vi "WSP2_InsertProcessDataWithFails.vi"(4 "Employee":string, 5 "FailString":string, 6 "EndTime":string, 7 "EntryTime":string, 8 "PassFail":i32, 9 "ProcessName":string, 10 "StationName":string, 11 "SerialNumber":string) -> (0 "error out":errorcluster, 3 "ReplyTrace":string)   [LabVIEW 2023]
uses:
  C:/Elatch-Bench-Test/VIs 64 bits/Elatch-Bench-Test/DLL/WSConnector.dll
  DLL/WSConnector.dll
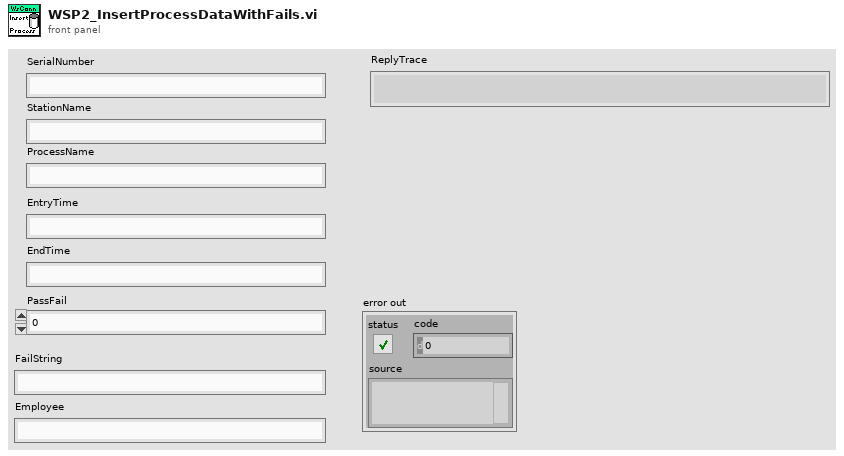
[diagram p1: front panel]
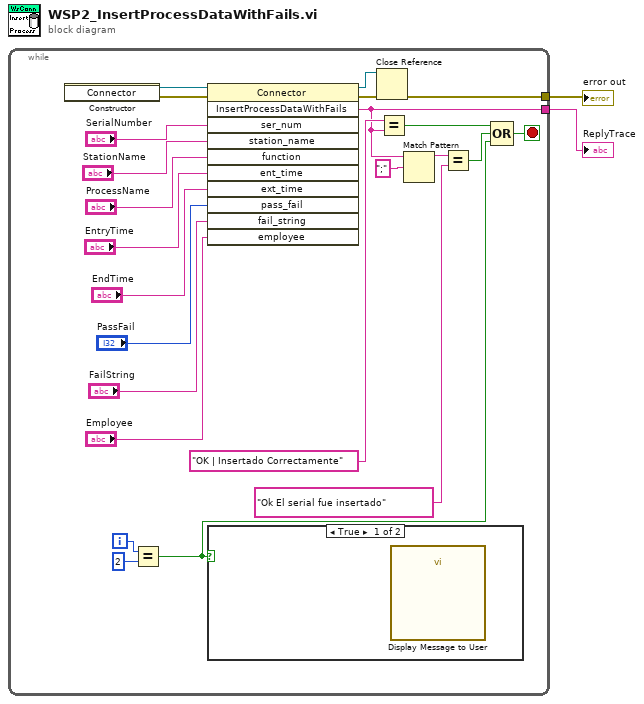
[diagram p0: block diagram]
diagram:
  n1 = while {
    tunnel: [w4] -> w2
    tunnel: [w3] -> w1
    i -> [w11]
    stop <- w9 stop-if-true
    n2 = constructor class="Connector"() -> (reference out=w18:refnum<k24>, error out=w7:errorcluster)  [unwired: 3 in, 1 out]
    n3 = Equal?(x=w11, y=2) -> (x = y?=w8:bool)
    n4 = invoke class="Connector" method="InsertProcessDataWithFails"(reference=w18, error in=w7, "ser_num"="SerialNumber", "station_name"="StationName", "function"="ProcessName", "ent_time"="EntryTime", "ext_time"="EndTime", "pass_fail"="PassFail", "fail_string"="FailString", "employee"="Employee") -> (reference out=w5:refnum<k24>, error out=w6:errorcluster, "InsertProcessDataWithFails"=w3:string)  [unwired: 1 in, 8 out]
    n5 = case shown="True" w8 {
      frame True {
        n6 = call "Display Message to User"() -> ()  [unwired: 10 in, 2 out]
      }
      frame False {
      }
    }
    n7 = Close Reference(reference=w5, error in (no error)=w6) -> (error out=w4:errorcluster)
    n8 = Equal?(x="OK | Insertado Correctamente", y=w3) -> (x = y?=w13:bool)
    n9 = Match Pattern(string=w3, regular expression=";") -> (before substring=w15:string)  [unwired: 1 in, 3 out]
    n10 = Equal?(x=w15, y="Ok El serial fue insertado") -> (x = y?=w14:bool)
    n11 = Compound Arithmetic op=OR(w13, w14, w8) -> (w9:bool)
  }
  "error out" <- w2
  "ReplyTrace" <- w1
